vi "Main.vi"() -> ()   [LabVIEW 2018]
uses:
  Clusters/FileDataChannel.ctl
  <vilib>/Platform/TimedLoop/XDataNode/timing_clust.ctl
  <vilib>/Platform/TimedLoop/XDataNode/nitl_modes.ctl
  <vilib>/Platform/TimedLoop/XDataNode/wakeup.ctl
  Clusters/SwapIndexes.ctl
  Clusters/SwapIn.ctl
  Clusters/RoscoParams.ctl
  Clusters/SimulationConstants.ctl
  <vilib>/platform/TimedLoop/XDataNode/XDataNode.xnode
  <vilib>/Platform/TimedLoop/XDataNode/XDNodeRunTimeDep.lvlib
panel:
  out "Generator Speed (rad/s)":sgl(slide)=7.06858e-05 scale=-4.0..4.0
  in  "?":enum32{"Scopes", "Extras"}(tab)
  out "Generator Speed":sgl(graph)
  out "Torque Setpoint (kNm)":sgl(graph)
  out "Pitch Setpoint":sgl(graph)
  in  "GenSpeed Mean":sgl=40.0
  in  "GenSpeeed Amplitude":sgl=20.0
  out "Rotor Speed (rad/s)":sgl(slide)=7.06858e-05 scale=-4.0..4.0
  out "Torque Setpoint (kNm)":sgl(knob) scale=0.0..21586451.0
  out "Pitch Setpoint":sgl(knob) scale=0.0..1.5
  out "Power (kW)":sgl(slide) scale=-15000.0..15000.0 scale format="%.2f"
  in  "Init WindSpeed(m/s)":sgl=7.0
  in  "File path":path=path "/home/lvuser/rosco-tests"
  out "SimLoop Late?":bool
  out "FIFO Loop Late?":bool
  in  "Base filename":string="rosco-tests"
  out "Writing to cRIO?":bool
  in  "WriteData":bool
  in  "?":T1
  out "#RT FIFO":u32
  out "Call to Rosco Failed?":bool
  out "Rosco Return Message":string
  in  "?":bool
  out "time(s)":dbl
  out "RT Loop Late?":bool
  # "FOCAL Realtime Control (IEA 15MW)"
  # "SENSOR INPUTS"
  # "FILEWRITING SETTINGS"
  # "ERRORS"
  # "TURBINE SPECIFICATIONS"
  # "ROSCO OUTPUTS"
  # "RATED POWER: 15000000 W"
  # "RATED TORQUE: 19624046.66 Nm"
  # "RATED GEN SPEED: 0.79168 rad/s"
  # "ROSCO INPUTS"
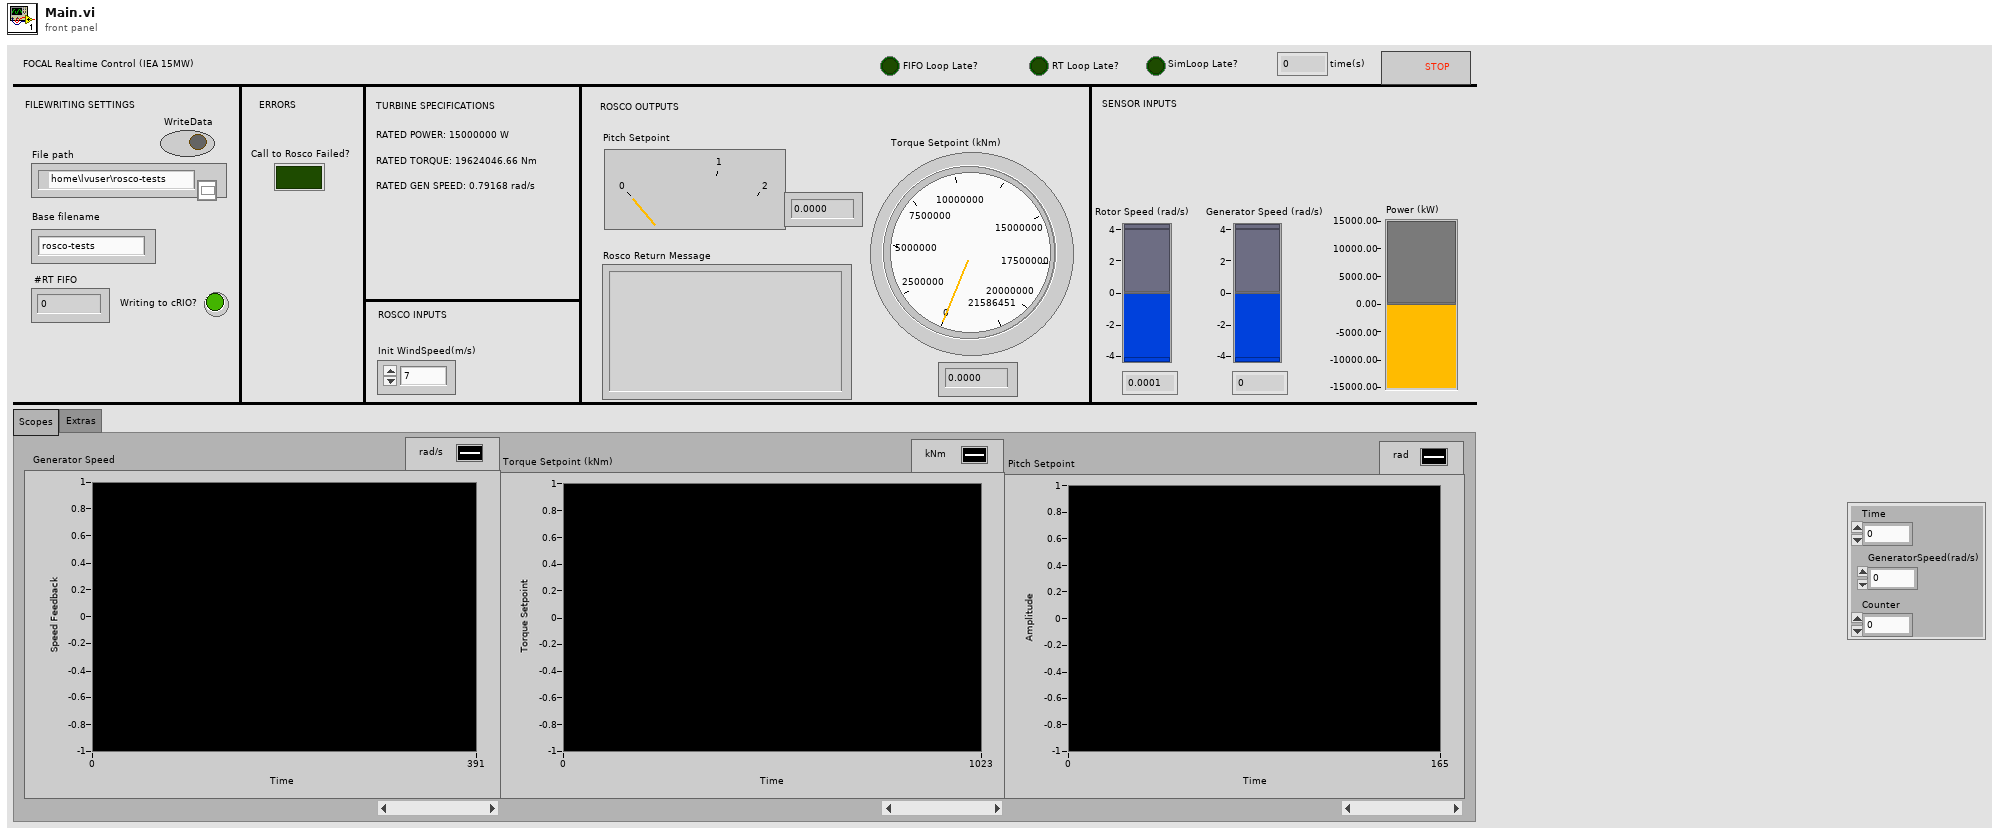
[diagram p1: front panel]
types:
  T1 = typedef "FileDataChannel.ctl" = cluster{"GeneratorSpeed(rad/s)":sgl, "Counter":sgl, "Time":sgl}
  T2 = typedef "SwapIndexes.ctl" = cluster{"iSTATUS":i32, "TIME":i32, "DT":i32, "BL_PITCH_1":i32, "VS_GENPWR":i32, "GEN_SPEED":i32, "ROT_SPEED":i32, "GENTQMEAS":i32, "Y_M":i32, "HORWINDV":i32, "ROOTMOOP1":i32, "ROOTMOOP2":i32, "BL_PITCH_2":i32, "BL_PITCH_3":i32, "ROOTMOOP3":i32, "INFILE_SIZE":i32, "FA_ACC":i32, "NUM_BLADES":i32, " OUT BL_PITCH":i32, "OUT_ TORQUE":i32, "OUTFILE_SIZE ":i32, "AVCMSG_SIZE":i32, "AERODYN TQ":i32}
  T3 = typedef "SwapIn.ctl" = cluster{"BladePitch(rad)":sgl, "RotorSpeed(rad/s)":sgl, "GeneratorSpeed(rad/s)":sgl, " GeneratorTorque(Nm)":sgl, " Generator Power(W) ":sgl, " WindSpeed(m/s)":sgl, "aviMSGLength":sgl, "InfileLength":sgl, "OutfileLength":sgl, "iStatus":sgl, "Time":sgl, "Dt":sgl, "NumberofBlades":sgl}
  T4 = typedef "RoscoParams.ctl" = cluster{"avrSWAP":sgl[], "aviFAIL":i32, "avcMSG":string, "ReturnValue":i32}
  T5 = typedef "XDNodeRunTimeDep.lvlib/timing_clust.ctl" = cluster{"Expected End [f-1]":u64, "Actual End [f-1]":u64, "Finished Late? [f-1]":bool, "Expected End [i-1]":u64, "Actual End [i-1]":u64, "Finished Late? [i-1]":bool, "Expected Start [i]":u64, "Actual Start [i]":u64, "Expected Start [f]":u64, "Actual Start [f]":u64, "Source Name":string, "Structure Name":string, "Period":i64, "Deadline":i64, "Offset":i64, "Start":i64, "Priority":i32, "Timeout":i32, "Mode":T6, "Wakeup Reason":T7, "Error":errorcluster, "Source Type":string, "Secondary Source Type":string, "Global End Time":u64, "Global Start Time":u64, "Frame Duration":u64, "Iteration Duration":u64, "Assigned CPU":i32, "I/O Scan Engine Mode":u32}
  T6 = typedef "XDNodeRunTimeDep.lvlib/nitl_modes.ctl" = enum32{"No Change", "Process missed periods, maintain original phase", "Discard missed periods, maintain original phase", "Process missed periods, ignore original phase", "Discard missed periods, ignore original phase"}
  T7 = typedef "XDNodeRunTimeDep.lvlib/wakeup.ctl" = enum32{"Normal", "Aborted", "Asynchronous wakeup", "Timing source error", "Timed loop error", "Timeout"}
  T8 = typedef "SimulationConstants.ctl" = cluster{"Ngear":sgl, "RotorInertia":sgl, "GeneratorEff":sgl}
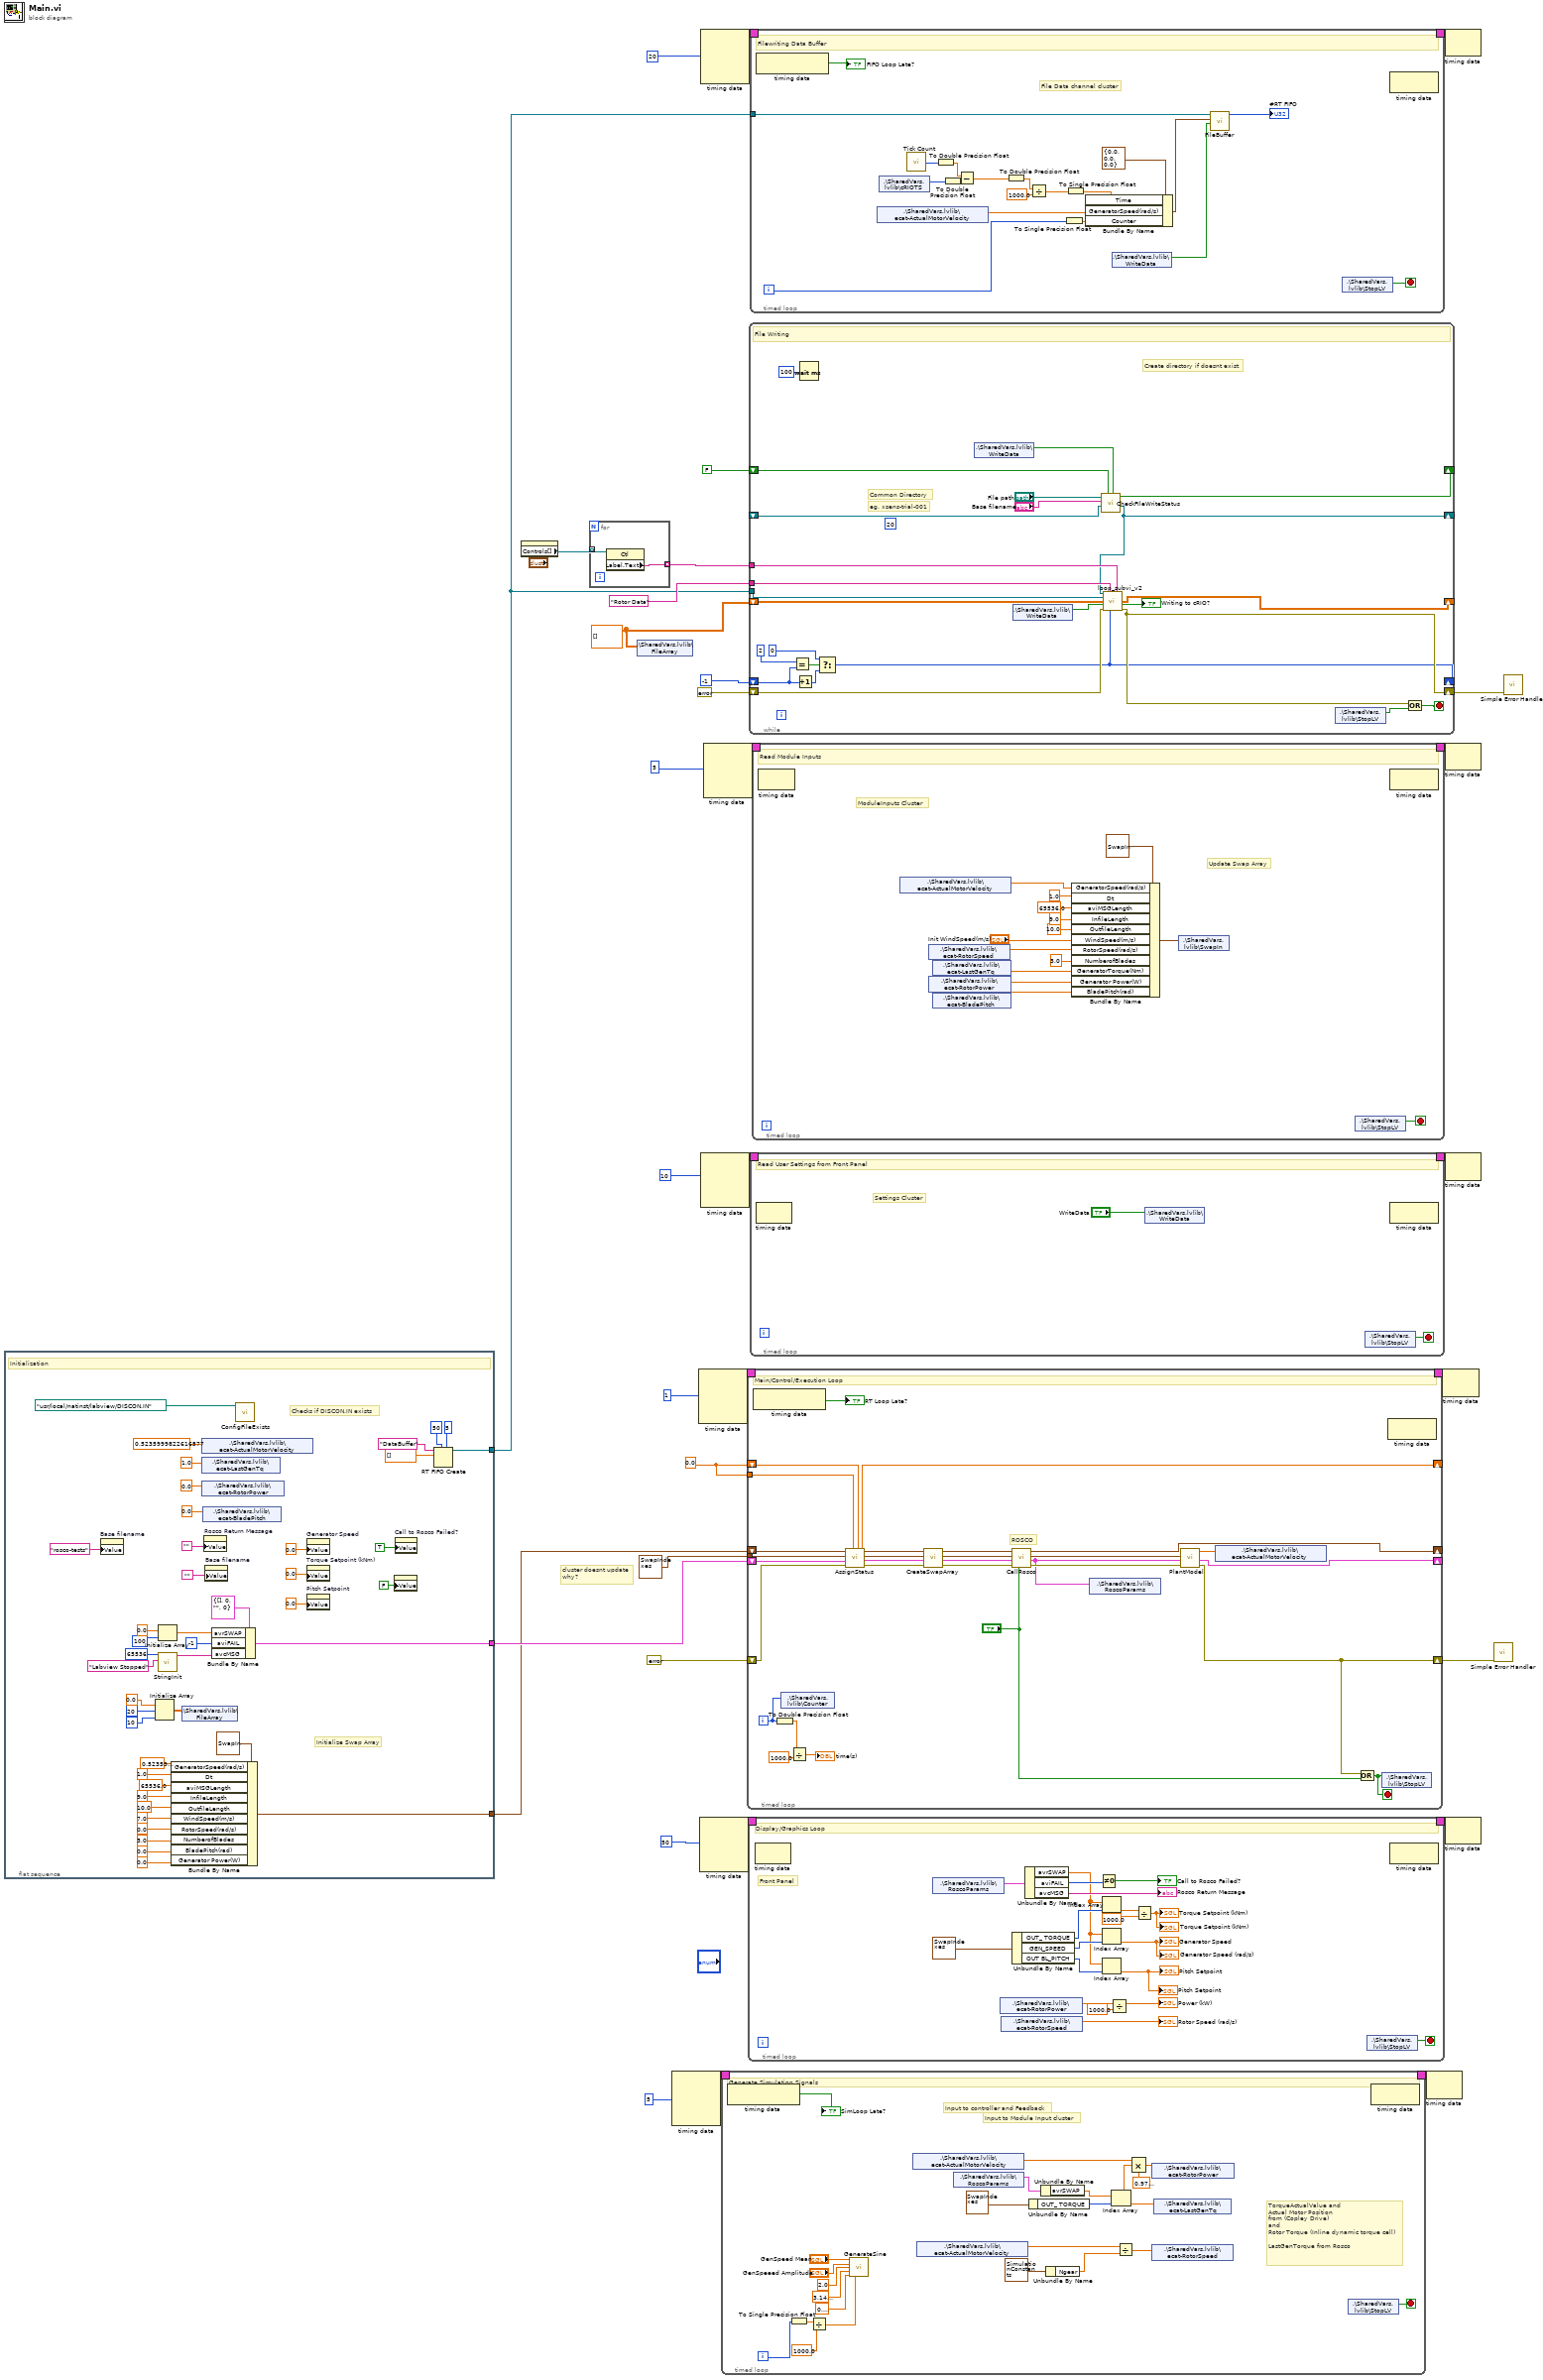
[diagram p0: block diagram]
diagram:
  w9 = dbl[][] [] ("File array 2")
  w17 = 0.0 ("y")
  (unwired) i64 20 ("Period")
  # "cluster doesnt update\nwhy?"
  n1 = flat-sequence {
    tunnel: [w69] -> w16
    tunnel: [w61] -> w10
    tunnel: [w37] -> w4
    frame #0 {
      # "Initialize Swap Array"
      # "Checks if DISCON.IN exists"
      # "Initialization"
      n2 = property on="Base filename" class="Str"("Value"="rosco-tests" ("Base filename")) -> ()  [unwired: 2 in, 2 out]
      n3 = Initialize Array(0.0 ("element"), 20 ("dimension size"), 10 ("dimension size")) -> (w57:dbl[][])
      n4 = Initialize Array(sgl 0.0 ("element"), 100 ("dimension size")) -> (w38:sgl[])
      n5 = call "StringInit.vi"("accOUTNAME"="Labview Stopped", "dimension size"=65536) -> ("result string"=w70:string)  [unwired: 9 in]
      n6 = Bundle By Name(cluster=T3 {"BladePitch(rad)"=0.0, "RotorSpeed(rad/s)"=0.0, "GeneratorSpeed(rad/s)"=0.0, " GeneratorTorque(Nm)"=0.0, " Generator Power(W) "=0.0, " WindSpeed(m/s)"=0.0, "aviMSGLength"=0.0, "InfileLength"=0.0, "OutfileLength"=0.0, "iStatus"=0.0, "Time"=0.0, "Dt"=0.0, "NumberofBlades"=0.0}, "GeneratorSpeed(rad/s)"=sgl 0.5236, "Dt"=sgl 1.0, "aviMSGLength"=sgl 65536.0 ("new element/subarray"), "InfileLength"=sgl 9.0 ("new element/subarray"), "OutfileLength"=sgl 10.0 ("new element/subarray"), "WindSpeed(m/s)"=sgl 7.0, "RotorSpeed(rad/s)"=sgl 0.0, "NumberofBlades"=sgl 3.0, "BladePitch(rad)"=sgl 0.0, "Generator Power(W)"=sgl 0.0) -> (w37:T3)
      n7 = shared-variable ".\\SharedVars.lvlib\\FileArray"(w57) -> ()  [unwired: 1 in, 1 out]
      n8 = shared-variable ".\\SharedVars.lvlib\\ecat-ActualMotorVelocity"(sgl 0.5236) -> ()  [unwired: 1 in, 1 out]
      n9 = shared-variable ".\\SharedVars.lvlib\\ecat-LastGenTq"(sgl 1.0 ("LastGenTq")) -> ()  [unwired: 1 in, 1 out]
      n10 = shared-variable ".\\SharedVars.lvlib\\ecat-RotorPower"(sgl 0.0 ("RotorPower")) -> ()  [unwired: 1 in, 1 out]
      n11 = shared-variable ".\\SharedVars.lvlib\\ecat-BladePitch"(sgl 0.0 ("BladePitch")) -> ()  [unwired: 1 in, 1 out]
      n12 = property on="Rosco Return Message" class="Str"("Value"="") -> ()  [unwired: 2 in, 2 out]
      n13 = property on="Base filename" class="Str"("Value"="") -> ()  [unwired: 2 in, 2 out]
      n14 = Bundle By Name(cluster=T4 {"avrSWAP"=[], "aviFAIL"=0, "avcMSG"="", "ReturnValue"=0}, "avrSWAP"=w38, "aviFAIL"=-1, "avcMSG"=w70) -> (w69:T4)
      n15 = call "ConfigFileExists.vi"("path"=path "/usr/local/natinst/labview/DISCON.IN") -> ()  [unwired: 11 in]
      n16 = property on="Generator Speed" class="WFChart (strict)"("Value"=sgl 0.0 ("Generator Speed")) -> ()  [unwired: 2 in, 2 out]
      n17 = property on="Torque Setpoint (kNm)" class="WFChart (strict)"("Value"=sgl 0.0 ("Generator Speed")) -> ()  [unwired: 2 in, 2 out]
      n18 = property on="Pitch Setpoint" class="WFChart (strict)"("Value"=sgl 0.0 ("Generator Speed")) -> ()  [unwired: 2 in, 2 out]
      n19 = property class="Bool (strict)"("Value"=FALSE) -> ()  [unwired: 2 in, 2 out]
      n20 = property on="Call to Rosco Failed?" class="Bool (strict)"("Value"=TRUE ("Call to Rosco Failed?")) -> ()  [unwired: 2 in, 2 out]
      n21 = RT FIFO Create(0:"DataBuffer" ("name (unnamed)"), 1:dbl[] [] ("appended array"), 4:u32 50, 6:u32 5) -> (8:w61:refnum<k33>)  [unwired: 4 in, 2 out]
    }
  }
  n22 = property class="Clust (strict)"() -> ("Controls[]"=w13:refnum<vi>[])  [unwired: 2 in, 2 out]
  n23 = for {
    tunnel: w13 -> [w78] mode=indexing
    tunnel: [w77] -> w12 mode=indexing
    n24 = property class="Ctl"(reference=w78) -> ("Label.Text"=w77:string)  [unwired: 1 in, 2 out]
  }
  n25 = shared-variable ".\\SharedVars.lvlib\\FileArray"(w9) -> ()  [unwired: 1 in, 1 out]
  n26 = node-c288(i64 5 ("Period")) -> (w25:T5)  [unwired: 3 in]
  n27 = node-c288(i64 1 ("Period")) -> (w23:T5)  [unwired: 3 in]
  n28 = node-c288(i64 50 ("Period")) -> (w27:T5)  [unwired: 3 in]
  n29 = node-c288(i64 20 ("Period")) -> (w33:T5)  [unwired: 3 in]
  n30 = node-c288(i64 10 ("Period")) -> (w29:T5)  [unwired: 3 in]
  n31 = node-c288(i64 5 ("Period")) -> (w31:T5)  [unwired: 3 in]
  n32 = timed-loop {
    timing: w25 -> [_]
    timing-out: [_] -> w24
    i -> [w99]
    stop <- w101 stop-if-true
    # "TorqueActualValue and \nActual Motor Position \nfrom (Copley Drive)\nand\nRotor Torque (Inline dynamic torque cell)\n\nLastGenTorque from Rosco"
    # "Input to Module Input cluster"
    # "Input to controller and Feedback"
    # "Generate Simulation Signals"
    n33 = node-c288() -> (→"SimLoop Late?":bool)  [unwired: 1 in]
    n34 = To Single Precision Float(number=w99) -> (single precision float=w100:sgl)
    n35 = Divide(x=w100, y=sgl 1000.0) -> (x/y=w93:sgl)
    n36 = call "GenerateSine.vi"("GenSpeed Mean"="GenSpeed Mean", "GenSpeeed Amplitude"="GenSpeeed Amplitude", "2"=sgl 2.0 ("value"), "pi"=sgl 3.14 ("value"), "frequency (f)"=sgl 0.1 ("value"), "time (s)"=w93) -> ()  [unwired: 9 in, 1 out]
    n37 = shared-variable ".\\SharedVars.lvlib\\ecat-ActualMotorVelocity"() -> (w86:sgl)  [unwired: 1 in, 1 out]
    n38 = shared-variable ".\\SharedVars.lvlib\\ecat-ActualMotorVelocity"() -> (w82:sgl)  [unwired: 1 in, 1 out]
    n39 = shared-variable ".\\SharedVars.lvlib\\RoscoParams"() -> (w85:T4)  [unwired: 1 in, 1 out]
    n40 = Unbundle By Name(T2 {"iSTATUS"=0, "TIME"=1, "DT"=2, "BL_PITCH_1"=3, "VS_GENPWR"=13, "GEN_SPEED"=19, "ROT_SPEED"=20, "GENTQMEAS"=22, "Y_M"=23, "HORWINDV"=26, "ROOTMOOP1"=29, "ROOTMOOP2"=30, "BL_PITCH_2"=32, "BL_PITCH_3"=33, "ROOTMOOP3"=31, "INFILE_SIZE"=49, "FA_ACC"=52, "NUM_BLADES"=60, " OUT BL_PITCH"=44, "OUT_ TORQUE"=46, "OUTFILE_SIZE "=50, "AVCMSG_SIZE"=48, "AERODYN TQ"=89} ("Index In")) -> ("OUT_ TORQUE"=w87:i32)
    n41 = Unbundle By Name(w85) -> ("avrSWAP"=w88:sgl[])
    n42 = Unbundle By Name(T8 {"Ngear"=1.0, "RotorInertia"=318628130.0, "GeneratorEff"=0.97} ("SimulationConst")) -> ("Ngear"=w80:sgl)
    n43 = Index Array(array=w88, index=w87) -> (element=w91:sgl)
    n44 = Divide(x=w82, y=w80) -> (x/y=w79:sgl)
    n45 = Compound Arithmetic op=MULTIPLY(w86, w91, sgl 0.97 ("value")) -> (w89:sgl)
    n46 = shared-variable ".\\SharedVars.lvlib\\ecat-RotorPower"(w89) -> ()  [unwired: 1 in, 1 out]
    n47 = shared-variable ".\\SharedVars.lvlib\\ecat-RotorSpeed"(w79) -> ()  [unwired: 1 in, 1 out]
    n48 = shared-variable ".\\SharedVars.lvlib\\ecat-LastGenTq"(w91) -> ()  [unwired: 1 in, 1 out]
    n49 = shared-variable ".\\SharedVars.lvlib\\StopLV"() -> (w101:bool)  [unwired: 1 in, 1 out]
    n50 = node-c288() -> ()  [unwired: 1 in, 1 out]
  }
  n51 = timed-loop {
    timing: w23 -> [_]
    timing-out: [_] -> w22
    shift-right: [w119] -> _
    shift-left: w17 -> [w121]
    tunnel: w17 -> [w120]
    tunnel: T2 {"iSTATUS"=0, "TIME"=1, "DT"=2, "BL_PITCH_1"=3, "VS_GENPWR"=13, "GEN_SPEED"=19, "ROT_SPEED"=20, "GENTQMEAS"=22, "Y_M"=23, "HORWINDV"=26, "ROOTMOOP1"=29, "ROOTMOOP2"=30, "BL_PITCH_2"=32, "BL_PITCH_3"=33, "ROOTMOOP3"=31, "INFILE_SIZE"=49, "FA_ACC"=52, "NUM_BLADES"=60, " OUT BL_PITCH"=44, "OUT_ TORQUE"=46, "OUTFILE_SIZE "=50, "AVCMSG_SIZE"=48, "AERODYN TQ"=89} ("Index In") -> [w126]
    shift-right: [w106] -> _
    shift-left: w16 -> [w125]
    shift-right: [w107] -> _
    shift-left: w4 -> [w116]
    shift-right: [w105] -> w2
    shift-left: errorcluster {"status"=FALSE, "code"=0, "source"=""} ("error out") -> [w113]
    i -> [w117]
    stop <- w111 stop-if-true
    # "ROSCO"
    # "Main/Control/Execution Loop"
    n52 = node-c288() -> (→"RT Loop Late?":bool)  [unwired: 1 in]
    n53 = To Double Precision Float(number=w117) -> (double precision float=w132:dbl)
    n54 = shared-variable ".\\SharedVars.lvlib\\Counter"(w117) -> ()  [unwired: 1 in, 1 out]
    n55 = Divide(x=w132, y=1000.0) -> (x/y=→"time(s)":dbl)
    n56 = call "AssignStatus.vi"("LoopCount"=w121, "Init Val"=w120, "error in (no error)"=w113, "ROSCO Params"=w125, 10:w126, "SwapIn"=w116) -> ("error out"=w129:errorcluster, "ROSCO Params 2"=w123:T4, 2:w124:T2, "SwapIn"=w128:T3, "Count+1"=w119:dbl)  [unwired: 1 in]
    n57 = call "CreateSwapArray.vi"("error in (no error)"=w129, "ROSCO Params"=w123, "Index In"=w124, "SwapIn"=w128) -> ("error out"=w122:errorcluster, "ROSCO Params Out"=w127:T4, "Index Out"=w114:T2, "SwapIn Out"=w115:T3)  [unwired: 4 in]
    n58 = call "CallRosco.vi"("StopLV"="?", "error in (no error)"=w122, "ROSCO Params in"=w127, 10:w114, "SwapIn"=w115) -> ("error out"=w110:errorcluster, "ROSCO Params out"=w109:T4, 2:w108:T2, "SwapIn"=w107:T3)  [unwired: 3 in]
    n59 = shared-variable ".\\SharedVars.lvlib\\RoscoParams"(w109) -> ()  [unwired: 1 in, 1 out]
    n60 = call "PlantModel.vi"("error in (no error)"=w110, "ROSCO Params in"=w109, 9:w108) -> ("error out"=w105:errorcluster, "ROSCO Params out"=w106:T4, "wdot/w"=w118:sgl)  [unwired: 5 in]
    n61 = shared-variable ".\\SharedVars.lvlib\\ecat-ActualMotorVelocity"(w118) -> ()  [unwired: 1 in, 1 out]
    n62 = Or(x=w105, y="?") -> (x .or. y?=w111:bool)
    n63 = shared-variable ".\\SharedVars.lvlib\\StopLV"(w111) -> ()  [unwired: 1 in, 1 out]
    n64 = node-c288() -> ()  [unwired: 1 in, 1 out]
  }
  n65 = timed-loop {
    timing: w27 -> [_]
    timing-out: [_] -> w26
    stop <- w155 stop-if-true
    # "Front Panel"
    # "Display/Graphics Loop"
    n66 = node-c288() -> ()  [unwired: 1 in, 1 out]
    n67 = shared-variable ".\\SharedVars.lvlib\\RoscoParams"() -> (w154:T4)  [unwired: 1 in, 1 out]
    n68 = shared-variable ".\\SharedVars.lvlib\\ecat-RotorPower"() -> (w143:sgl)  [unwired: 1 in, 1 out]
    n69 = shared-variable ".\\SharedVars.lvlib\\ecat-RotorSpeed"() -> (→"Rotor Speed (rad/s)":sgl)  [unwired: 1 in, 1 out]
    n70 = Unbundle By Name(T2 {"iSTATUS"=0, "TIME"=1, "DT"=2, "BL_PITCH_1"=3, "VS_GENPWR"=13, "GEN_SPEED"=19, "ROT_SPEED"=20, "GENTQMEAS"=22, "Y_M"=23, "HORWINDV"=26, "ROOTMOOP1"=29, "ROOTMOOP2"=30, "BL_PITCH_2"=32, "BL_PITCH_3"=33, "ROOTMOOP3"=31, "INFILE_SIZE"=49, "FA_ACC"=52, "NUM_BLADES"=60, " OUT BL_PITCH"=44, "OUT_ TORQUE"=46, "OUTFILE_SIZE "=49, "AVCMSG_SIZE"=49, "AERODYN TQ"=46}) -> ("OUT_ TORQUE"=w152:i32, "GEN_SPEED"=w151:i32, "OUT BL_PITCH"=w145:i32)
    n71 = Unbundle By Name(w154) -> ("avrSWAP"=w146:sgl[], "aviFAIL"=w149:i32, "avcMSG"=→"Rosco Return Message":string)
    n72 = Not Equal To 0?(x=w149) -> (x != 0?=→"Call to Rosco Failed?":bool)
    n73 = Index Array(array=w146, index=w152) -> (element=w147:sgl)
    n74 = Index Array(array=w146, index=w151) -> (element=→"Generator Speed" →"Generator Speed (rad/s)":sgl)
    n75 = Index Array(array=w146, index=w145) -> (element=→"Pitch Setpoint" →"Pitch Setpoint":sgl)
    n76 = Divide(x=w143, y=sgl 1000.0) -> (x/y=→"Power (kW)":sgl)
    n77 = Divide(x=w147, y=sgl 1000.0) -> (x/y=→"Torque Setpoint (kNm)" →"Torque Setpoint (kNm)":sgl)
    n78 = shared-variable ".\\SharedVars.lvlib\\StopLV"() -> (w155:bool)  [unwired: 1 in, 1 out]
    n79 = node-c288() -> ()  [unwired: 1 in, 1 out]
  }
  n80 = while {
    shift-right: [w158] -> _
    shift-left: _ -> [w159]
    shift-right: [w166] -> _
    shift-left: FALSE -> [w167]
    shift-right: [w179] -> w5
    shift-left: errorcluster {"status"=FALSE, "code"=0, "source"=""} ("error out") -> [w178]
    tunnel: "Rotor Data" -> [w161]
    tunnel: w12 -> [w162]
    tunnel: w10 -> [w163]
    shift-right: [w175] -> _
    shift-left: -1 -> [w177]
    shift-right: [w170] -> _
    shift-left: w9 -> [w176]
    stop <- w181 stop-if-true
    # "eg. xsens-trial-001"
    # "Create directory if doesnt exist"
    # "Common Directory"
    # "File Writing"
    n81 = Equal?(x=2 ("t"), y=w177) -> (x = y?=w172:bool)
    n82 = Increment(x=w177) -> (x+1=w171:i32)
    n83 = Wait (ms)(milliseconds to wait=u32 100) -> ()  [unwired: 1 out]
    n84 = Select(t=0, s=w172, f=w171) -> (s? t:f=w175:i32)
    n85 = shared-variable ".\\SharedVars.lvlib\\WriteData"() -> (w168:bool)  [unwired: 1 in, 1 out]
    n86 = shared-variable ".\\SharedVars.lvlib\\WriteData"() -> (w164:bool)  [unwired: 1 in, 1 out]
    n87 = call "CheckFIleWriteStatus.vi"("WriteDataButtonVal"=w168, "WritePrevVal"=w167, "Refnum in"=w159, "Base filename"="Base filename", "File path"="File path") -> ("Refnum out"=w158:refnum<k34>, "WriteCurrentVal"=w166:bool)  [unwired: 5 in]
    n88 = call "loop_subvi_v2.vi"("Refnum in"=w158, "Group Name"=w161, "Channel Names"=w162, "rt fifo"=w163, "File array"=w176, "Write?"=w164, "error in (no error)"=w178, "index"=w175) -> ("File array 2"=w170:dbl[][], "Writing to file"=→"Writing to cRIO?":bool, "error out"=w179:errorcluster)  [unwired: 4 in, 1 out]
    n89 = shared-variable ".\\SharedVars.lvlib\\StopLV"() -> (w182:bool)  [unwired: 1 in, 1 out]
    n90 = Or(x=w179, y=w182) -> (x .or. y?=w181:bool)
  }
  n91 = timed-loop {
    timing: w33 -> [_]
    timing-out: [_] -> w32
    tunnel: w10 -> [w189]
    i -> [w184]
    stop <- w201 stop-if-true
    # "File Data channel cluster"
    # "Filewriting Data Buffer"
    n92 = node-c288() -> (→"FIFO Loop Late?":bool)  [unwired: 1 in]
    n93 = shared-variable ".\\SharedVars.lvlib\\ecat-ActualMotorVelocity"() -> (w194:sgl)  [unwired: 1 in, 1 out]
    n94 = shared-variable ".\\SharedVars.lvlib\\cRIOTS"() -> (w196:u64)  [unwired: 1 in, 1 out]
    n95 = call "Tick Count"() -> ("Tick Count(mSec)"=w197:u32)
    n96 = To Double Precision Float(number=w197) -> (double precision float=w186:dbl)
    n97 = To Double Precision Float(number=w196) -> (double precision float=w195:dbl)
    n98 = Subtract(x=w186, y=w195) -> (x-y=w198:dbl)
    n99 = To Double Precision Float(number=w198) -> (double precision float=w200:dbl)
    n100 = Divide(x=w200, y=1000.0) -> (x/y=w185:dbl)
    n101 = To Single Precision Float(number=w184) -> (single precision float=w187:sgl)
    n102 = To Single Precision Float(number=w185) -> (single precision float=w193:sgl)
    n103 = Bundle By Name(cluster=T1 {"GeneratorSpeed(rad/s)"=0.0, "Counter"=0.0, "Time"=0.0} ("SwapIn"), "Time"=w193, "GeneratorSpeed(rad/s)"=w194, "Counter"=w187) -> (w191:T1)
    n104 = shared-variable ".\\SharedVars.lvlib\\WriteData"() -> (w190:bool)  [unwired: 1 in, 1 out]
    n105 = call "FileBuffer.vi"("Boolean"=w190, "FileDataChannel"=w191, "Refnum in"=w189) -> ("# elements"=→"#RT FIFO":u32)  [unwired: 8 in]
    n106 = shared-variable ".\\SharedVars.lvlib\\StopLV"() -> (w201:bool)  [unwired: 1 in, 1 out]
    n107 = node-c288() -> ()  [unwired: 1 in, 1 out]
  }
  n108 = timed-loop {
    timing: w29 -> [_]
    timing-out: [_] -> w28
    stop <- w206 stop-if-true
    # "Settings Cluster"
    # "Read User Settings from Front Panel"
    n109 = node-c288() -> ()  [unwired: 1 in, 1 out]
    n110 = shared-variable ".\\SharedVars.lvlib\\WriteData"("WriteData") -> ()  [unwired: 1 in, 1 out]
    n111 = shared-variable ".\\SharedVars.lvlib\\StopLV"() -> (w206:bool)  [unwired: 1 in, 1 out]
    n112 = node-c288() -> ()  [unwired: 1 in, 1 out]
  }
  n113 = timed-loop {
    timing: w31 -> [_]
    timing-out: [_] -> w30
    stop <- w222 stop-if-true
    # "Update Swap Array"
    # "ModuleInputs Cluster"
    # "Read Module Inputs"
    n114 = node-c288() -> ()  [unwired: 1 in, 1 out]
    n115 = shared-variable ".\\SharedVars.lvlib\\ecat-ActualMotorVelocity"() -> (w214:sgl)  [unwired: 1 in, 1 out]
    n116 = shared-variable ".\\SharedVars.lvlib\\ecat-RotorSpeed"() -> (w209:sgl)  [unwired: 1 in, 1 out]
    n117 = shared-variable ".\\SharedVars.lvlib\\ecat-RotorPower"() -> (w211:sgl)  [unwired: 1 in, 1 out]
    n118 = shared-variable ".\\SharedVars.lvlib\\ecat-BladePitch"() -> (w210:sgl)  [unwired: 1 in, 1 out]
    n119 = shared-variable ".\\SharedVars.lvlib\\ecat-LastGenTq"() -> (w212:sgl)  [unwired: 1 in, 1 out]
    n120 = Bundle By Name(cluster=T3 {"BladePitch(rad)"=0.0, "RotorSpeed(rad/s)"=0.0, "GeneratorSpeed(rad/s)"=0.0, " GeneratorTorque(Nm)"=0.0, " Generator Power(W) "=0.0, " WindSpeed(m/s)"=0.0, "aviMSGLength"=0.0, "InfileLength"=0.0, "OutfileLength"=0.0, "iStatus"=0.0, "Time"=0.0, "Dt"=0.0, "NumberofBlades"=0.0}, "GeneratorSpeed(rad/s)"=w214, "Dt"=sgl 1.0, "aviMSGLength"=sgl 65536.0 ("new element/subarray"), "InfileLength"=sgl 9.0 ("new element/subarray"), "OutfileLength"=sgl 10.0 ("new element/subarray"), "WindSpeed(m/s)"="Init WindSpeed(m/s)", "RotorSpeed(rad/s)"=w209, "NumberofBlades"=sgl 3.0, "GeneratorTorque(Nm)"=w212, "Generator Power(W)"=w211, "BladePitch(rad)"=w210) -> (w221:T3)
    n121 = shared-variable ".\\SharedVars.lvlib\\SwapIn"(w221) -> ()  [unwired: 1 in, 1 out]
    n122 = shared-variable ".\\SharedVars.lvlib\\StopLV"() -> (w222:bool)  [unwired: 1 in, 1 out]
    n123 = node-c288() -> ()  [unwired: 1 in, 1 out]
  }
  n124 = node-c288(w24) -> ()  [unwired: 1 out]
  n125 = node-c288(w22) -> ()  [unwired: 1 out]
  n126 = node-c288(w32) -> ()  [unwired: 1 out]
  n127 = node-c288(w30) -> ()  [unwired: 1 out]
  n128 = node-c288(w28) -> ()  [unwired: 1 out]
  n129 = node-c288(w26) -> ()  [unwired: 1 out]
  n130 = call <vilib>:"Simple Error Handler.vi"("error in (no error)"=w2) -> ()  [unwired: 4 in, 5 out]
  n131 = call <vilib>:"Simple Error Handler.vi"("error in (no error)"=w5) -> ()  [unwired: 4 in, 5 out]
